vi "Main.vi"(11 "Module Admin":refnum<class "Delacor_lib_QMH_Module Admin.lvclass">) -> ()   [LabVIEW 2019, in "HMI.lvlib"]
doc: "This template is based off of the Queued Message Handler design pattern and the Queued Message Handler project template that ships with LabVIEW.\n\nThe main difference is that the queue is private to this module and communication between modules is performed via Broadcast and Request events.\n\nRequest events are wrapped in public API methods and are handled in the Event Handling Loop (EHL) of this VI. Any module can register for Broadcast events sent by this module. The EHL generates messages based on user interface actions.\n\nThe Message Handling Loop (MHL) processes messages generated by the EHL, or by other messages. The messages are string values, so new messages can be added easily to the Message Cases case structure in the MHL. Each message cluster can also provide an optional value for Message Data, which is a variant that can be converted to whatever message-specific data is required.\n_____\nBased on DQMH Dev Tools: Project Template 7.1.2.1547."
uses:
  HMI.lvlib
  <vilib>/Delacor/Delacor QMH/Libraries/Module Admin_class/Delacor_lib_QMH_Module Admin.lvclass
  Module Data--cluster.ctl
  Stop Argument--cluster.ctl
  <vilib>/Delacor/Delacor QMH/Libraries/Message Queue_class/Delacor_lib_QMH_Message Queue.lvclass/Delacor_lib_QMH_Message Queue.ctl
  <vilib>/Delacor/Delacor QMH/Libraries/Module Admin_class/Delacor_lib_QMH_Module Admin.lvclass/Delacor_lib_QMH_Module Admin.ctl
  Open UDP Connection Argument--cluster.ctl
  <vilib>/Utility/miscctls.llb/LVPointTypeDef.ctl
  <vilib>/Delacor/Delacor QMH/Libraries/Message Queue_class/Delacor_lib_QMH_Enqueue Message (Single).vi
  <vilib>/Delacor/Delacor QMH/Libraries/Module Admin_class/Delacor_lib_QMH_Get External Launch.vi
  <vilib>/Delacor/Delacor QMH/Libraries/Message Queue_class/Delacor_lib_QMH_Message Queue.lvclass
panel:
  out "Analog Input":dbl[](array[numeric])
  out "Digital Input":bool[](array[boolean])
  out "error out":errorcluster
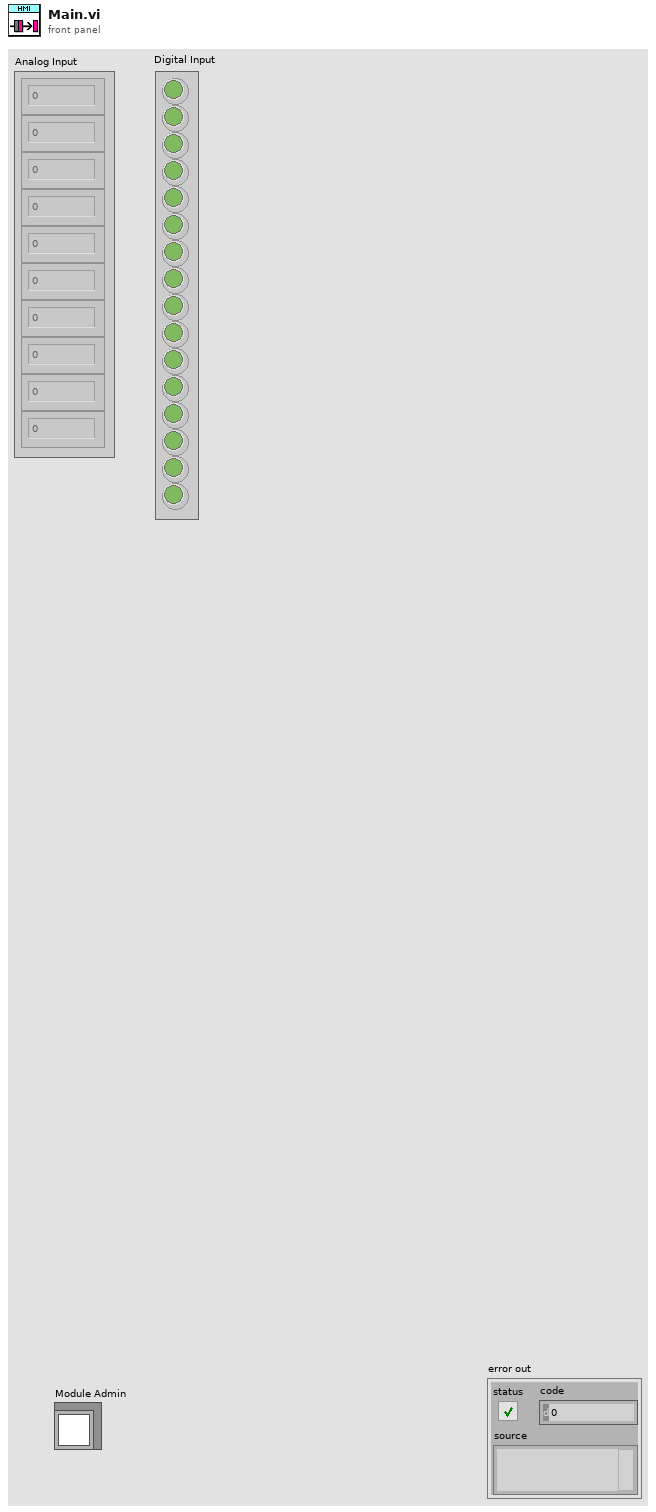
[diagram p1: front panel]
types:
  T1 = typedef "HMI.lvlib/Request Events--cluster.ctl" = cluster{"Stop Module":refnum<user-event>, "Show Panel":refnum<user-event>, "Hide Panel":refnum<user-event>, "Get Module Execution Status":refnum<user-event>, "Show Diagram":refnum<user-event>, "Private.Open UDP Connection":refnum<user-event>, "Private.Get UDP Info":refnum<user-event>}
  T2 = typedef "HMI.lvlib/Module Data--cluster.ctl" = cluster{"Status":string, "IP RT":string, "Port RT":u16, "Port Host":u16, "connection ID":refnum<k16>}
  T3 = enum32{"invalid lock state", "Not Locked", "Locked (No Password)", "Password-protected"}
  T4 = typedef "HMI.lvlib/Stop Argument--cluster.ctl" = cluster{"Origin":string, "Exit via Stop Module Req?":bool, "Wait for Module to stop?":bool}
  T5 = typedef "HMI.lvlib/Open UDP Connection Argument--cluster.ctl" = cluster{"Boolean":bool}
  T6 = typedef "LVPointTypeDef.ctl" = cluster{"Horizontal":i16, "Vertical":i16}
  T7 = enum32{"Invalid", "Standard", "Closed", "Hidden", "Minimized", "Maximized"}
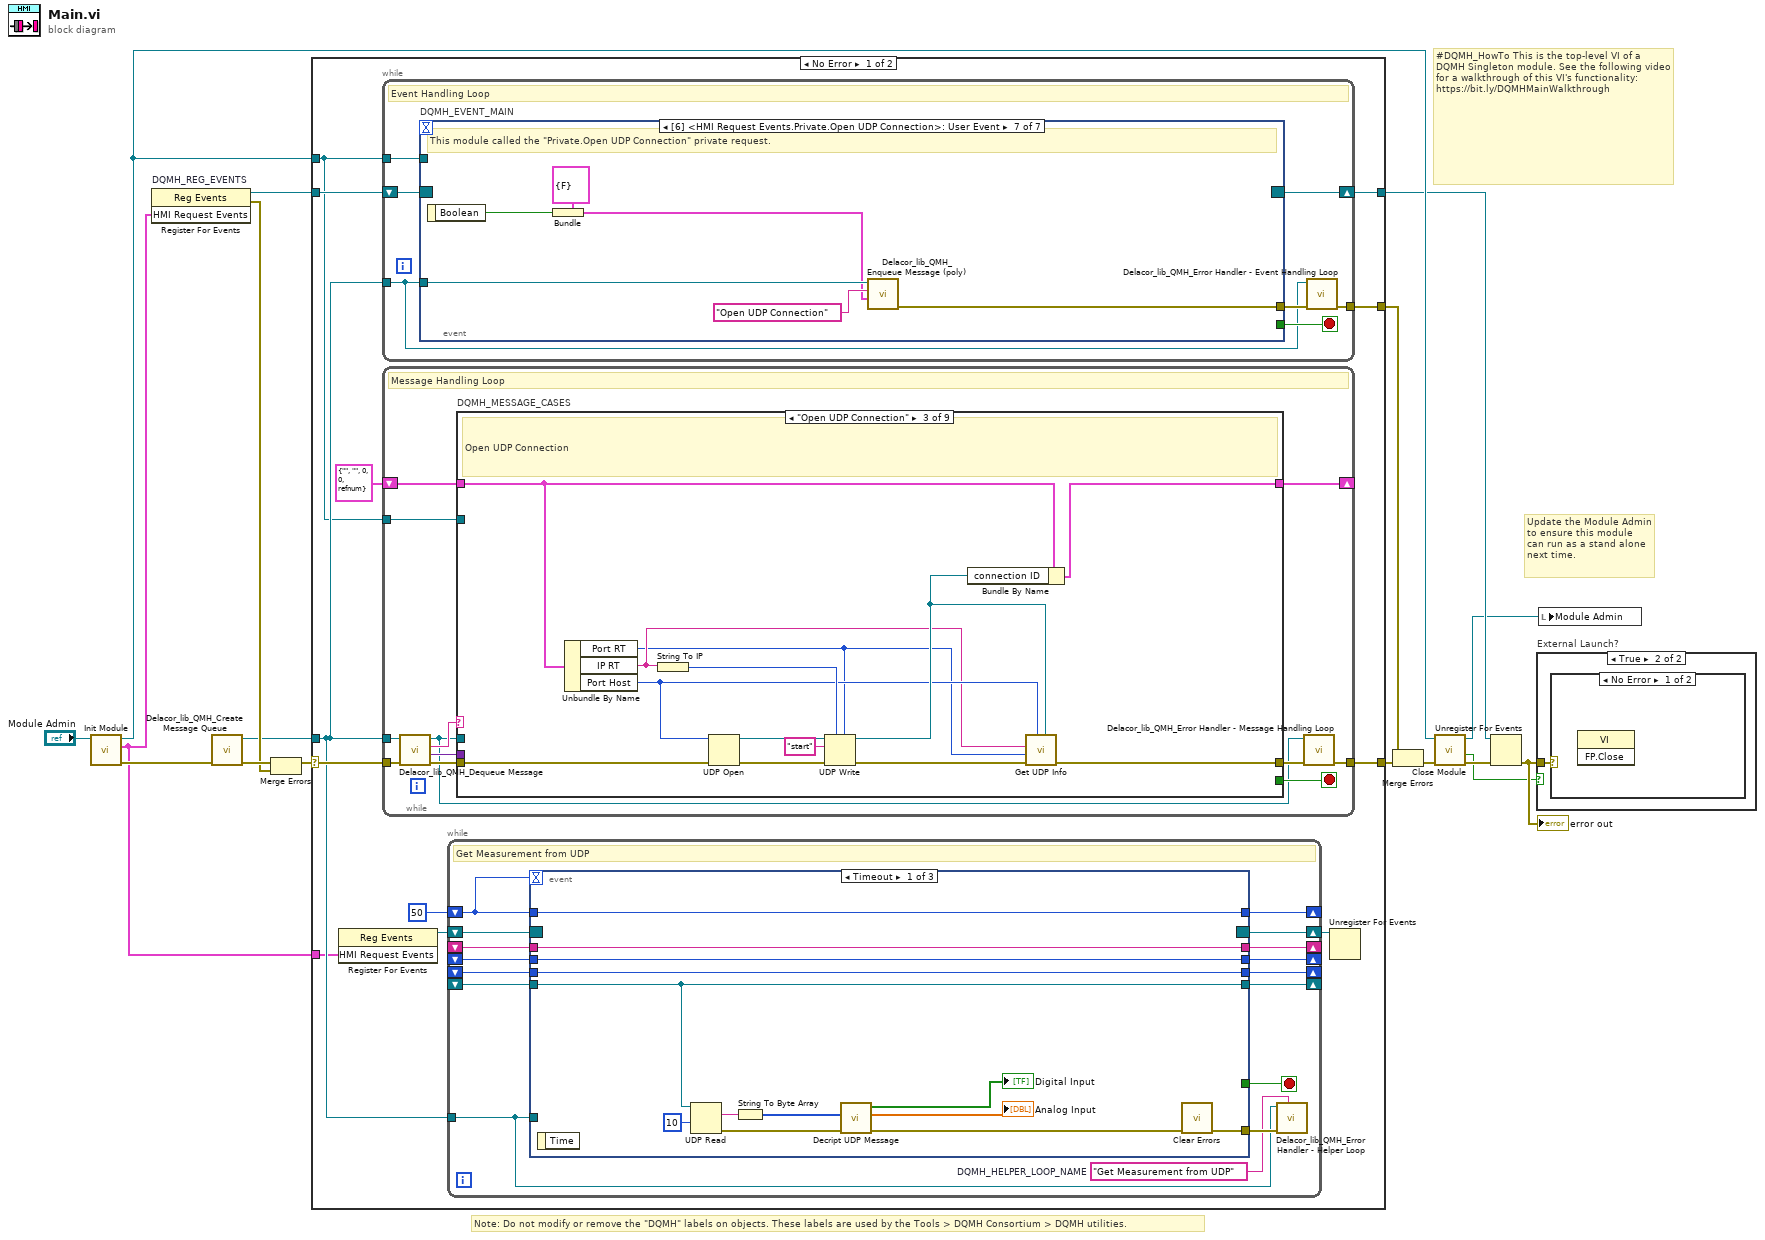
[diagram p0: block diagram]
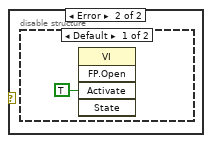
[diagram p3: hidden frame]
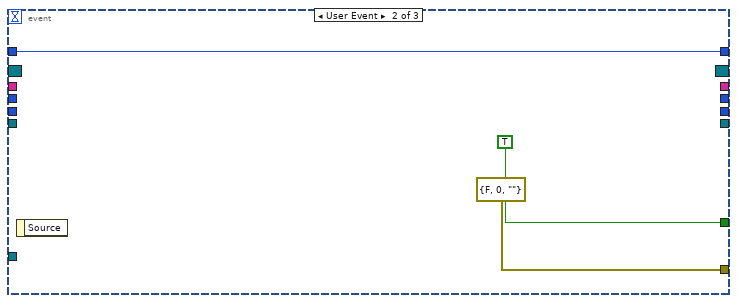
[diagram p5: hidden frame]
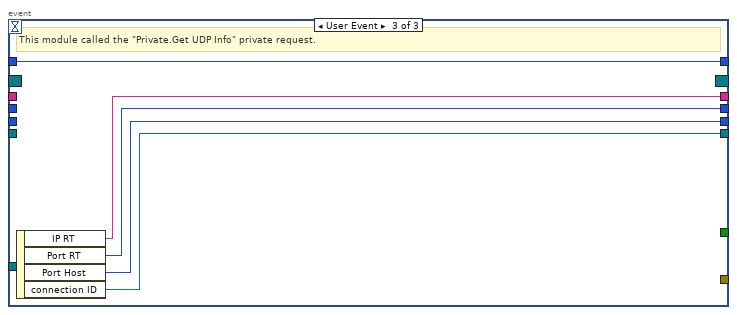
[diagram p6: hidden frame]
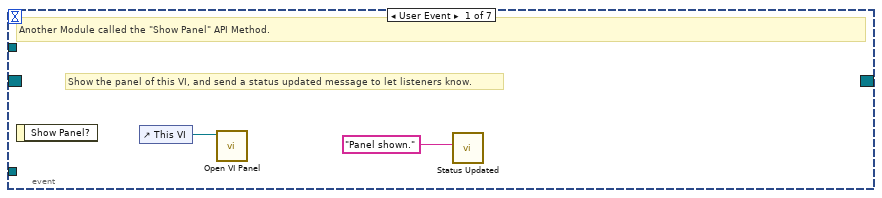
[diagram p7: hidden frame]
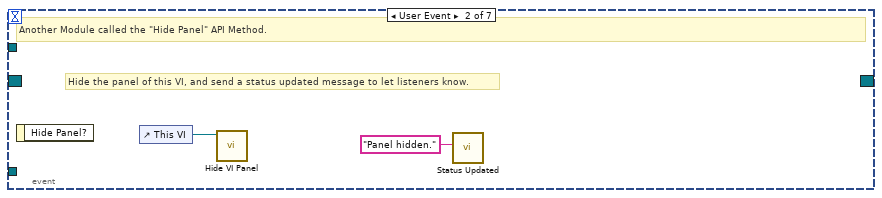
[diagram p8: hidden frame]
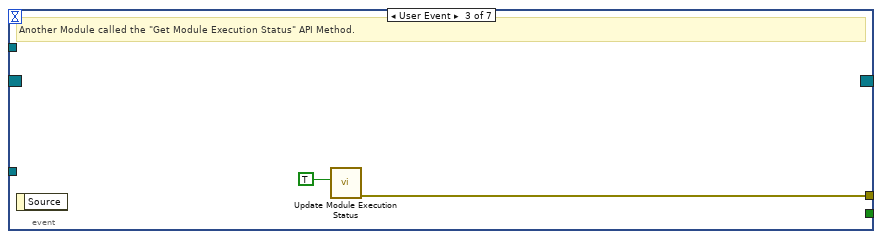
[diagram p9: hidden frame]
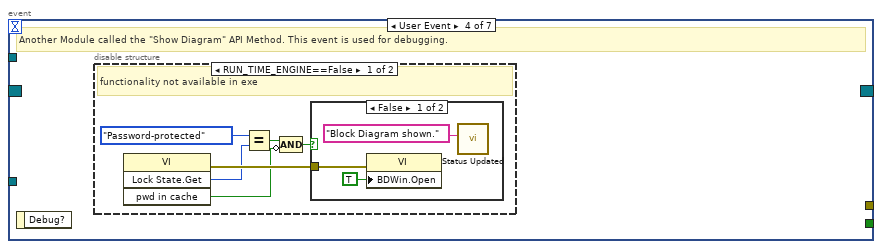
[diagram p10: hidden frame]
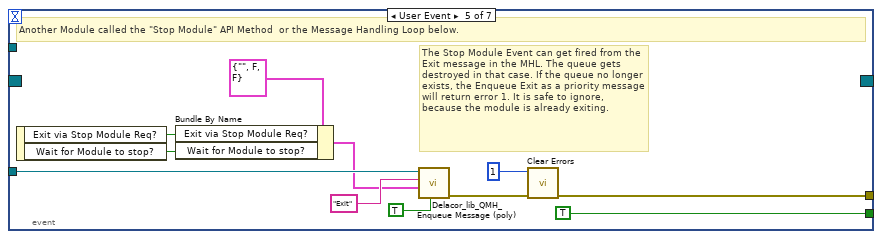
[diagram p13: hidden frame]
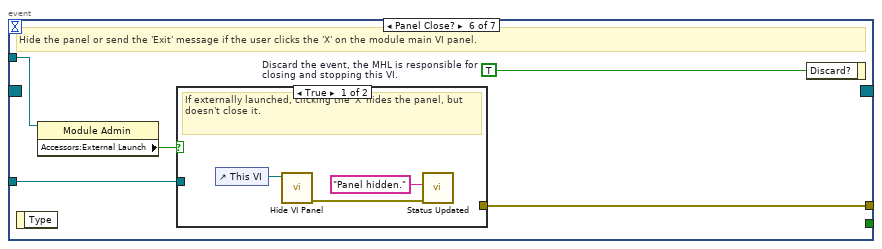
[diagram p14: hidden frame]
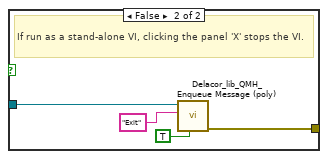
[diagram p15: hidden frame]
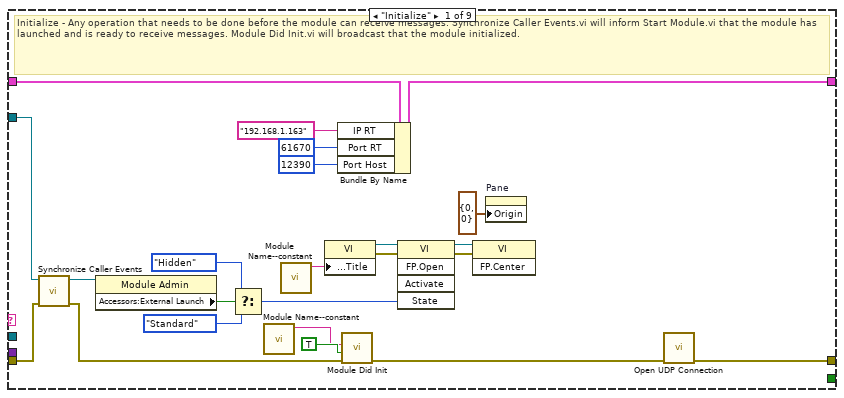
[diagram p16: hidden frame]
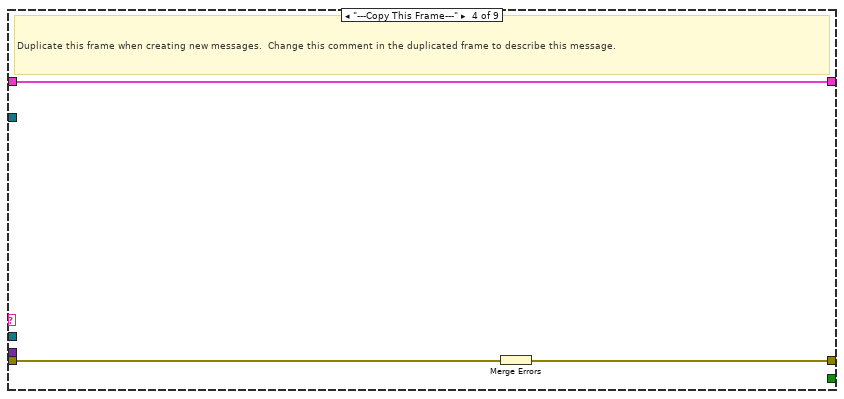
[diagram p18: hidden frame]
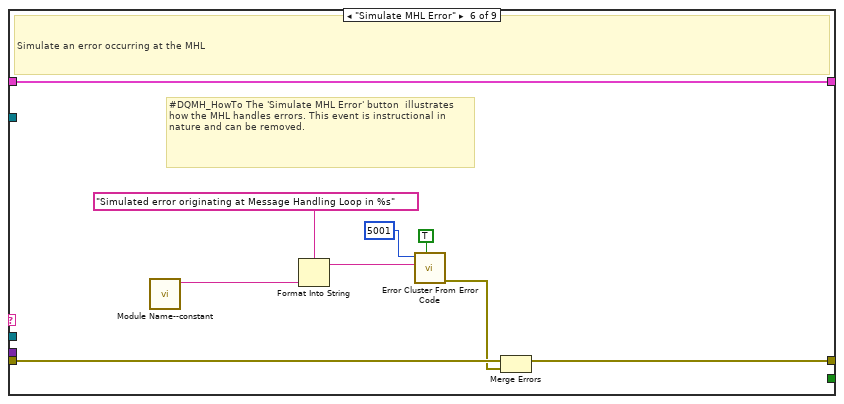
[diagram p20: hidden frame]
diagram:
  # "#DQMH_HowTo This is the top-level VI of a DQMH Singleton module. See the following video for a walkthrough of this VI's functionality: https://bit.ly/DQMHMainWalkthrough"
  # "Note: Do not modify or remove the \"DQMH\" labels on objects. These labels are used by the Tools > DQMH Consortium > DQMH utilities."
  # "Update the Module Admin to ensure this module can run as a stand alone next time."
  n1 = call "Init Module.vi"("Singleton Module Admin in"="Module Admin") -> ("error out"=w16:errorcluster, "HMI Request Events"=w1:T1, "Singleton Module Admin out"=w8:refnum<class "Delacor_lib_QMH_Module Admin.lvclass">)  [unwired: 8 in]
  n2 = register-events "DQMH_REG_EVENTS"(w1) -> (reference out=w6:refnum<event-registration>, error out=w9:errorcluster)  [unwired: 2 in]
  n3 = call <vilib>:"Delacor_lib_QMH_Create Message Queue.vi"("error in"=w16) -> ("error out"=w11:errorcluster, "Message Queue"=w5:refnum<class "Delacor_lib_QMH_Message Queue.lvclass">)  [unwired: 9 in]
  n4 = Merge Errors(w11, w9) -> (w10:errorcluster)
  n5 = case shown="No Error" w10 {
    selector: w10 -> [w27 w231]
    tunnel: [w29 w230] -> w17
    tunnel: [w26 w229] -> w7
    tunnel: w6 -> [w24 w229]
    tunnel: w5 -> [w23 w224]
    tunnel: [w28 _] -> w14
    tunnel: w8 -> [w22 w225]
    tunnel: w1 -> [w21 _]
    frame No Error {
      n6 = register-events ("DQMH_HELPER_REGFOREVENTS")(w21) -> (reference out=w19:refnum<event-registration>)  [unwired: 2 in, 1 out]
      n7 = while {
        tunnel: w23 -> [w67]
        shift-right: [w70] -> w26
        shift-left: w24 -> [w71]
        tunnel: [w72] -> w28
        tunnel: w22 -> [w68]
        stop <- w69 stop-if-true
        # "Event Handling Loop"
        n8 = event "DQMH_EVENT_MAIN" shown="[6] <HMI Request Events.Private.Open UDP Connection>: User Event" {
          selector: w71 -> [_ _ _ _ _ _ _]
          dyn-events: [_ _ _ _ _ _ _] -> w70
          timeout: _ -> [_ _ _ _ _ _ _]
          tunnel: [_ _ _ _ TRUE ("Discard?") _ _] -> w69
          tunnel: w67 -> [_ _ _ _ w95 w102 w117]
          tunnel: [_ _ w79 _ w98 w104 w112] -> w73
          tunnel: w68 -> [_ _ _ _ _ w101 _]
          event User Event {
            # "Show the panel of this VI, and send a status updated message to let listeners know."
            # "Another Module called the \"Show Panel\" API Method."
            n9 = event-data() -> ()  [unwired: 1 in, 1 out]
            n10 = control-ref of="This VI"() -> (w75:refnum<vi>)
            n11 = call "Open VI Panel.vi"("VI"=w75) -> ()  [unwired: 10 in, 1 out]
            n12 = call "Status Updated.vi"("Status"="Panel shown." ("format string")) -> ()  [unwired: 10 in, 1 out]
          }
          event User Event {
            # "Hide the panel of this VI, and send a status updated message to let listeners know."
            # "Another Module called the \"Hide Panel\" API Method."
            n13 = event-data() -> ()  [unwired: 1 in, 1 out]
            n14 = control-ref of="This VI"() -> (w77:refnum<vi>)
            n15 = call "Hide VI Panel.vi"("VI"=w77) -> ()  [unwired: 10 in, 1 out]
            n16 = call "Status Updated.vi"("Status"="Panel hidden." ("format string")) -> ()  [unwired: 10 in, 1 out]
          }
          event User Event {
            # "Another Module called the \"Get Module Execution Status\" API Method."
            n17 = event-data() -> ()  [unwired: 1 in, 1 out]
            n18 = call "Update Module Execution Status.vi"("Running?"=TRUE) -> ("error out"=w79:errorcluster)  [unwired: 10 in]
          }
          event User Event {
            # "Another Module called the \"Show Diagram\" API Method. This event is used for debugging."
            n19 = event-data() -> ()  [unwired: 1 in, 1 out]
            n20 = disable-structure shown="RUN_TIME_ENGINE==False" {
              frame condition #0 (active) {
                # "functionality not available in exe"
                n21 = invoke on="Invoke Node" class="VI" method="Lock State.Get"() -> (error out=w85:errorcluster, "Get Lock State"=w84:T3, "pwd in cache"=w81:bool)  [unwired: 4 in, 1 out]
                n22 = Equal?(x=T3."Password-protected", y=w84) -> (x = y?=w82:bool)
                n23 = Compound Arithmetic op=AND(w82, invert w81) -> (w80:bool)
                n24 = case shown="False" w80 {
                  tunnel: w85 -> [w88 _]
                  frame False {
                    n25 = property on="Property Node" class="VI"(error in=w88, "BDWin.Open"=TRUE ("Block Diagram Window:Open")) -> ()  [unwired: 1 in, 2 out]
                    n26 = call "Status Updated.vi"("Status"="Block Diagram shown." ("format string")) -> ()  [unwired: 10 in, 1 out]
                  }
                  frame True {
                    # "Password-protected VI, and the password is not in the cache. Do not show the diagram."
                  }
                }
              }
              frame condition #1 {
              }
            }
          }
          event User Event {
            # "The Stop Module Event can get fired from the Exit message in the MHL. The queue gets destroyed in that case. If the queue no longer exists, the Enqueue Exit as a priority message will return error 1. It is safe to ignore, because the module is already exiting."
            # "Another Module called the \"Stop Module\" API Method  or the Message Handling Loop below."
            n27 = event-data() -> ("Exit via Stop Module Req?"=w91:bool, "Wait for Module to stop?"=w90:bool)  [unwired: 1 in]
            n28 = Bundle By Name(cluster=T4 {"Origin"="", "Exit via Stop Module Req?"=FALSE, "Wait for Module to stop?"=FALSE} ("Stop Argument"), "Exit via Stop Module Req?"=w91, "Wait for Module to stop?"=w90) -> (w89:T4)
            n29 = call-poly <vilib>:"Delacor_lib_QMH_Enqueue Message (poly).vi"("Priority Message? (F)"=TRUE, "Message Data"=w89, "Message"="Exit", "Message Queue in"=w95) -> ("error out"=w99:errorcluster)  [unwired: 6 in, 1 out]
            n30 = call <vilib>:"Clear Errors.vi"("error in (no error)"=w99, "specific error code to clear (0: all)"=1) -> ("error out"=w98:errorcluster)  [unwired: 4 in, 1 out]
          }
          event Panel Close? {
            w103 = TRUE  # Discard the event, the MHL is responsible for closing and stopping this VI.
            # "Hide the panel or send the 'Exit' message if the user clicks the 'X' on the module main VI panel."
            n31 = event-data() -> ()  [unwired: 1 in, 1 out]
            n32 = property on="Property Node" class="Module Admin"(reference=w101) -> ("Accessors:External Launch"=w100:bool)  [unwired: 1 in, 2 out]
            n33 = case shown="True" w100 {
              tunnel: w102 -> [_ w110]
              tunnel: [_ w111] -> w104
              frame True {
                # "If externally launched, clicking the 'X' hides the panel, but doesn't close it."
                n34 = control-ref of="This VI"() -> (w107:refnum<vi>)
                n35 = call "Hide VI Panel.vi"("VI"=w107) -> ("error out"=w105:errorcluster)  [unwired: 10 in]
                n36 = call "Status Updated.vi"("error in"=w105, "Status"="Panel hidden." ("format string")) -> ()  [unwired: 9 in, 1 out]
              }
              frame False {
                # "If run as a stand-alone VI, clicking the panel 'X' stops the VI."
                n37 = call-poly <vilib>:"Delacor_lib_QMH_Enqueue Message (poly).vi"("Priority Message? (F)"=TRUE, "Message"="Exit", "Message Queue in"=w110) -> ("error out"=w111:errorcluster)  [unwired: 7 in, 1 out]
              }
            }
            n38 = event-data ("Event Filter Node")("Discard?"=w103) -> ()  [unwired: 1 in, 1 out]
          }
          event User Event {
            # "This module called the \"Private.Open UDP Connection\" private request."
            n39 = event-data() -> ("Boolean"=w113:bool)  [unwired: 1 in]
            n40 = Bundle(cluster=T5 {"Boolean"=FALSE} ("Open UDP Connection Argument"), "Boolean"=w113) -> (w114:T5)
            n41 = call-poly <vilib>:"Delacor_lib_QMH_Enqueue Message (poly).vi"("Message Data"=w114, "Message"="Open UDP Connection", "Message Queue in"=w117) -> ("error out"=w112:errorcluster)  [unwired: 7 in, 1 out]
          }
        }
        n42 = call-dynamic "Delacor_lib_QMH_Error Handler - Event Handling Loop.vi"("error in"=w73, "Message Queue in"=w67) -> ("dup error in"=w72:errorcluster)  [unwired: 8 in, 1 out]
      }
      n43 = while {
        tunnel: w23 -> [w118]
        shift-right: [w126] -> _
        shift-left: T2 {"Status"="", "IP RT"="", "Port RT"=0, "Port Host"=0, "connection ID"=refnum} ("Data Cluster") -> [w127]
        tunnel: w27 -> [w129]
        tunnel: [w121] -> w29
        tunnel: w22 -> [w122]
        stop <- w125 stop-if-true
        # "Message Handling Loop"
        n44 = call-dynamic "Delacor_lib_QMH_Dequeue Message.vi"("error in"=w129, "Message Queue in"=w118) -> ("error out"=w128:errorcluster, "Message Data"=w123:variant, "Message"=w124:string, "Message Queue out"=w119:refnum<class "Delacor_lib_QMH_Message Queue.lvclass">)  [unwired: 6 in]
        n45 = case "DQMH_MESSAGE_CASES" shown="\"Open UDP Connection\"" w124 {
          selector: w124 -> [_ _ _ _ _ _ _ _ w219]
          tunnel: w119 -> [_ _ _ _ _ _ w185 w207 _]
          tunnel: w128 -> [w150 w154 w167 w170 w172 w181 w192 w213 w222]
          tunnel: [w135 w154 w159 w169 w172 w180 w188 w208 w223] -> w120
          tunnel: w127 -> [w133 w153 w164 w168 w171 w178 w187 w206 w220]
          tunnel: [w134 w153 w165 w168 w171 w178 w187 w206 w220] -> w126
          tunnel: [_ _ _ _ _ _ _ w205 _] -> w125
          tunnel: w123 -> [_ _ _ _ _ _ w186 w204 _]
          tunnel: w122 -> [w141 _ _ _ _ _ w184 w199 _]
          frame "Initialize" {
            # "Initialize - Any operation that needs to be done before the module can receive messages. Synchronize Caller Events.vi will inform Start Module.vi that the module has launched and is ready to receive messages. Module Did Init.vi will broadcast that the module initialized."
            n46 = call "Synchronize Caller Events.vi"("error in"=w150, "Singleton Module Admin in"=w141) -> ("error out"=w149:errorcluster, "Singleton Module Admin out"=w138:refnum<class "Delacor_lib_QMH_Module Admin.lvclass">)  [unwired: 8 in]
            n47 = property on="Property Node" class="Module Admin"(reference=w138) -> ("Accessors:External Launch"=w145:bool)  [unwired: 1 in, 2 out]
            n48 = Select(t=T7."Hidden" ("State"), s=w145, f=T7."Standard" ("State")) -> (s? t:f=w142:T7)
            n49 = call "Module Name--constant.vi"() -> ("Module Name"=w139:string)  [unwired: 11 in]
            n50 = call "Module Name--constant.vi"() -> ("Module Name"=w148:string)  [unwired: 11 in]
            n51 = property on="Property Node" class="VI"("Front Panel.Title"=w148) -> (reference out=w147:refnum<vi>, error out=w152:errorcluster)  [unwired: 2 in]
            n52 = Bundle By Name(cluster=w133, "IP RT"="192.168.1.163", "Port RT"=u16 61670, "Port Host"=u16 12390) -> (w134:T2)
            n53 = call "Module Did Init.vi"("error in"=w149, "Initialized?"=TRUE, "Origin"=w139) -> ("error out"=w136:errorcluster)  [unwired: 8 in]
            n54 = invoke on="Invoke Node" class="VI" method="FP.Open"(reference=w147, error in=w152, "State"=w142) -> (reference out=w146:refnum<vi>, error out=w151:errorcluster)  [unwired: 2 in, 3 out]
            n55 = invoke on="Invoke Node" class="VI" method="FP.Center"(reference=w146, error in=w151) -> ()  [unwired: 1 in, 3 out]
            n56 = property on="Pane" class="Pane"("Origin"=T6 {"Horizontal"=0, "Vertical"=0}) -> ()  [unwired: 2 in, 2 out]
            n57 = call "Open UDP Connection.vi"("error in"=w136) -> ("error out"=w135:errorcluster)  [unwired: 10 in]
          }
          frame "---Module Specific---" {
            # "Separator -- The following cases handle messages specific to this Module."
          }
          frame "Open UDP Connection" {
            # "Open UDP Connection"
            n58 = Unbundle By Name(w164) -> ("Port RT"=w155:u16, "IP RT"=w156:string, "Port Host"=w157:u16)
            n59 = String To IP(1:w156) -> (0:w161:u32)
            n60 = UDP Open(8:w167, 11:w157) -> (port=w163:refnum<k16>, 0:w166:errorcluster)  [unwired: 3 in, 1 out]
            n61 = UDP Write(address=w161, port or service name=w155, connection ID=w163, data in="start", 8:w166) -> (error out=w160:errorcluster, 3:w158:refnum<k16>)  [unwired: 1 in]
            n62 = Bundle By Name(cluster=w164, "connection ID"=w158) -> (w165:T2)
            n63 = call "Get UDP Info.vi"("connection ID"=w158, "Port Host"=w157, "error in"=w160, "Port RT"=w155, "IP RT"=w156) -> ("error out"=w159:errorcluster)  [unwired: 6 in]
          }
          frame "---Copy This Frame---" {
            # "Duplicate this frame when creating new messages.  Change this comment in the duplicated frame to describe this message."
            n64 = Merge Errors(w170) -> (w169:errorcluster)
          }
          frame "---Exit and Error Handling---" {
            # "Separator - The following cases handle errors and exit messages."
          }
          frame "Simulate MHL Error" {
            # "#DQMH_HowTo The 'Simulate MHL Error' button  illustrates how the MHL handles errors. This event is instructional in nature and can be removed."
            # "Simulate an error occurring at the MHL"
            n65 = call "Module Name--constant.vi"() -> ("Module Name"=w174:string)  [unwired: 11 in]
            n66 = Format Into String(format string="Simulated error originating at Message Handling Loop in %s", w174) -> (resulting string=w175:string)  [unwired: 2 in, 1 out]
            n67 = call <vilib>:"Error Cluster From Error Code.vi"("show call chain? (False)"=TRUE, "error message (\"\")"=w175, "error code (0)"=5001) -> ("error out"=w179:errorcluster)  [unwired: 6 in]
            n68 = Merge Errors(w181, w179) -> (w180:errorcluster)
          }
          frame "Error" {
            # "#DQMH_CodeRecommended - If the module is running in standalone mode (External Launch = FALSE), this code will pop up an error dialog and call the 'Exit' message if an error occurs. Add more fine-grained error management here."
            # "Error - Check the error message data and respond accordingly. This message is sent by the \"Error Handler\" VIs at the end of each loop in this application."
            n69 = property on="Property Node" class="Module Admin"(reference=w184) -> ("Accessors:External Launch"=w183:bool)  [unwired: 1 in, 2 out]
            n70 = Variant To Data(error in=w192, type=errorcluster {"status"=FALSE, "code"=0, "source"=""} ("error constant"), Variant=w186) -> (data=w182:errorcluster, error out=w190:errorcluster)
            n71 = local write "error out"(w182) -> ()
            n72 = call "Error Reported.vi"("Error"=w182) -> ()  [unwired: 10 in, 1 out]
            n73 = case shown="False" w183 {
              tunnel: [w197 _] -> w189
              tunnel: w185 -> [w195 _]
              tunnel: w182 -> [w196 _]
              frame False {
                n74 = disable-structure shown="Default" {
                  disable-tunnel: w196 -> [w198 _]
                  frame condition #0 (active) {
                    # "If the module is running standalone, then pop up an error dialog and call the \"Exit\" message."
                    n75 = call <vilib>:"Simple Error Handler.vi"("error in (no error)"=w198) -> ()  [unwired: 4 in, 5 out]
                  }
                  frame condition #1 {
                    # "To prevent the Simple Error Handler VI from being loaded (e.g. when deploying to a Real-Time target), add the Conditional Disable Symbol \"DQMH_Disable_SEH\" to your project and set it to TRUE."
                  }
                }
                n76 = call-poly <vilib>:"Delacor_lib_QMH_Enqueue Message (poly).vi"("Priority Message? (F)"=TRUE, "Message"="Exit", "Message Queue in"=w195) -> ("error out"=w197:errorcluster)  [unwired: 7 in, 1 out]
              }
              frame True {
                # "If the module was launched externally, calling the Error Reported broadcast VI is the only action performed by the \"Error\" message. The module's caller can then process the error appropriately."
              }
            }
            n77 = Merge Errors(w190, w189) -> (w188:errorcluster)
          }
          frame "Exit" {
            w203 = 91  # 91: not all Exit messages will have an argument
            w205 = TRUE  # Stop the VI
            # "Release the message queue reference"
            # "#DQMH_CodeNeeded - Add any required cleanup code here."
            # "Exit - Exit the application."
            n78 = Variant To Data(error in=w213, type=T4 {"Origin"="", "Exit via Stop Module Req?"=FALSE, "Wait for Module to stop?"=FALSE} ("Stop Argument"), Variant=w204) -> (data=w201:T4, error out=w210:errorcluster)
            n79 = call <vilib>:"Clear Errors.vi"("error in (no error)"=w210, "specific error code to clear (0: all)"=w203) -> ("error out"=w212:errorcluster)  [unwired: 4 in, 1 out]
            n80 = control-ref of="This VI"() -> (w200:refnum<vi>)
            n81 = call-dynamic "Delacor_lib_QMH_Release Message Queue.vi"("error in"=w212, "Message Queue"=w207) -> ("error out"=w211:errorcluster)  [unwired: 9 in]
            n82 = call "Handle Exit.vi"("Stop Argument"=w201, "Admin in"=w199, "VI reference"=w200) -> ("error out"=w209:errorcluster)  [unwired: 7 in, 1 out]
            n83 = Merge Errors(w211, w209) -> (w208:errorcluster)
            n84 = call "Error Reported.vi"("Error"=w208) -> ()  [unwired: 10 in, 1 out]
          }
          frame Default {
            # "'Default' case only runs if there is a message that isn't defined in any of the other cases.  Output a programming error."
            n85 = call "Module Name--constant.vi"() -> ("Module Name"=w218:string)  [unwired: 11 in]
            n86 = Format Into String(format string="The invalid message string \"%s\" was received in the Message Handling Loop for module \"%s\".", w219, w218) -> (resulting string=w214:string)  [unwired: 2 in, 1 out]
            n87 = call <vilib>:"Error Cluster From Error Code.vi"("show call chain? (False)"=TRUE, "error message (\"\")"=w214, "error code (0)"=1) -> ("error out"=w221:errorcluster)  [unwired: 6 in]
            n88 = Merge Errors(w222, w221) -> (w223:errorcluster)
          }
        }
        n89 = call-dynamic "Delacor_lib_QMH_Error Handler - Message Handling Loop.vi"("error in"=w120, "Message Queue in"=w119) -> ("dup error in"=w121:errorcluster)  [unwired: 8 in, 1 out]
      }
      n90 = while "DQMH_HELPER_LOOP" {
        shift-right: [w45] -> _
        shift-left: 50 -> [w44]
        shift-right: [w42] -> w20
        shift-left: w19 -> [w43]
        tunnel: w23 -> [w39]
        shift-right: [w37] -> _
        shift-left: _ -> [w36]
        shift-right: [w35] -> _
        shift-left: _ -> [w34]
        shift-right: [w33] -> _
        shift-left: _ -> [w32]
        shift-right: [w31] -> _
        shift-left: _ -> [w30]
        stop <- w41 stop-if-true
        w38 = "Get Measurement from UDP"  # DQMH_HELPER_LOOP_NAME
        # "Get Measurement from UDP"
        n91 = event "DQMH_HELPER_EVENT_STRUCTURE" shown="[0] Timeout" {
          selector: w43 -> [_ _ _]
          dyn-events: [_ _ _] -> w42
          timeout: w44 -> [_ _ _]
          tunnel: w44 -> [w58 w61 w66]
          tunnel: [w58 w61 w66] -> w45
          tunnel: [_ TRUE _] -> w41
          tunnel: [w51 errorcluster {"status"=FALSE, "code"=0, "source"=""} ("error constant") _] -> w40
          tunnel: w39 -> [_ _ _]
          tunnel: [w55 _ w65] -> w37
          tunnel: w36 -> [w55 _ _]
          tunnel: [w54 _ w64] -> w35
          tunnel: w34 -> [w54 _ _]
          tunnel: [w53 _ w63] -> w33
          tunnel: w32 -> [w53 _ _]
          tunnel: [w52 _ w62] -> w31
          tunnel: w30 -> [w52 _ _]
          event Timeout {
            n92 = event-data() -> ()  [unwired: 1 in, 1 out]
            n93 = UDP Read(connection ID=w52, timeout ms (25000)=10) -> (data out=w56:string, error out=w49:errorcluster)  [unwired: 2 in, 3 out]
            n94 = String To Byte Array(string=w56) -> (unsigned byte array=w50:u8[])
            n95 = call "Decript UDP Message.vi"("Error In"=w49, "UDP Message"=w50) -> ("Error Out"=w48:errorcluster, "Analog Input"=→"Analog Input":dbl[], "Digital Input"=→"Digital Input":bool[])  [unwired: 7 in]
            n96 = call <vilib>:"Clear Errors.vi"("error in (no error)"=w48) -> ("error out"=w51:errorcluster)  [unwired: 5 in, 1 out]
          }
          event User Event {
            n97 = event-data() -> ()  [unwired: 1 in, 1 out]
          }
          event User Event {
            # "This module called the \"Private.Get UDP Info\" private request."
            n98 = event-data() -> ("IP RT"=w65:string, "Port RT"=w64:u16, "Port Host"=w63:u16, "connection ID"=w62:refnum<k16>)  [unwired: 1 in]
          }
        }
        n99 = call-dynamic "Delacor_lib_QMH_Error Handler - Helper Loop.vi"("Error Debug"=w38, "error in"=w40, "Message Queue in"=w39) -> ()  [unwired: 7 in, 2 out]
      }
      n100 = Unregister For Events(event registration refnum=w20) -> ()  [unwired: 1 in, 1 out]
    }
    frame Error {
      # "Synchronize Caller Events.vi will inform Start Module.vi that the module has launched and will let the code calling Start Module.vi register for broadcasts and would permit the caller receive the broadcast that an error occurred at launch time."
      n101 = call-dynamic "Delacor_lib_QMH_Release Message Queue.vi"("error in"=w231, "Message Queue"=w224) -> ("error out"=w230:errorcluster)  [unwired: 9 in]
      n102 = call "Synchronize Caller Events.vi"("Singleton Module Admin in"=w225) -> ("error out"=w232:errorcluster)  [unwired: 9 in, 1 out]
      n103 = call "Module Name--constant.vi"() -> ("Module Name"=w228:string)  [unwired: 11 in]
      n104 = Format Into String(format string="An error occurred during initialization. %s is no longer running.", w228) -> (resulting string=w226:string)  [unwired: 2 in, 1 out]
      n105 = Merge Errors(w230, w232) -> (w233:errorcluster)
      n106 = call "Error Reported.vi"("Additional Information"=w226, "Error"=w233) -> ()  [unwired: 9 in, 1 out]
    }
  }
  n107 = Merge Errors(w14, w17) -> (w13:errorcluster)
  n108 = call "Close Module.vi"("error in"=w13, "Module Admin in"=w8) -> ("error out"=w15:errorcluster, "External Launch"=w2:bool, "Module Admin out"=w3:refnum<class "Delacor_lib_QMH_Module Admin.lvclass">)  [unwired: 7 in]
  n109 = Unregister For Events(event registration refnum=w7, error in=w15) -> (error out=w12:errorcluster)
  "error out" <- w12
  n110 = case "External Launch?" shown="True" w2 {
    tunnel: w12 -> [_ w234]
    frame False {
    }
    frame True {
      n111 = case shown="No Error" w234 {
        frame No Error {
          n112 = invoke on="Invoke Node" class="VI" method="FP.Close"() -> ()  [unwired: 3 in, 3 out]
        }
        frame Error {
          n113 = disable-structure shown="Default" {
            frame condition #0 (active) {
              n114 = invoke class="VI" method="FP.Open"("Activate"=TRUE ("Activate?")) -> ()  [unwired: 4 in, 5 out]
            }
            frame condition #1 {
              # "Don't show panel on error if running inside a built EXE."
            }
          }
        }
      }
    }
  }
  n115 = local write "Module Admin"(w3) -> ()
